vi "SLSC Scripting Constants.vi"() -> ()   [LabVIEW 2020, in "SLSC Switch Scripting.lvlib"]
doc: "Use this Global VI to access the GUIDs assigned to the page resources of the Custom Device."
uses:
  SLSC Switch Scripting.lvlib
panel:
  in  "Tab Control":T1(tab)=enum."Properties"
  in  "SLSC Sw:Status Section":string="Status"
  in  "SLSC Sw:Endpoint Section":string="Endpoint Configuration"
  in  "SLSC Sw:Prop:Reservation Group":string="Reservation Group"
  in  "SLSC Sw:Prop:Slot #":string="Slot #"
  in  "SLSC Sw:Prop:Model":string="Model"
  in  "SLSC Sw:Prop:Topology":string="Topology"
  in  "SLSC Sw:Prop:Switches JSON":string="Capabilities"
  in  "Compiled.Settings":string="Compiled.Settings"
  in  "GUID.SLSC Chassis":string="2d230194-1f79-4241-ad00-e5b0a0d634cb"
  in  "GUID.Status":string="fafe2633-52e8-4be6-bb95-b07e42834d60"
  in  "ChanList.HeartbeatChan":string="Heartbeat"
  in  "ChanList.StatusCode":string="Status code"
  in  "Desc.HeartbeatChan":string="Running count used for debugging. If this channel continues to increment, the custom device is still executing."
  in  "Desc.StatusCode":string="Status code of the custom device. A negative value indicates failure. A positive value indicates warning."
  in  "Paths.CDXML":path=path "SLSC Plugins/Modules/SLSC Switch/SLSC Module SLSC Switch.xml"
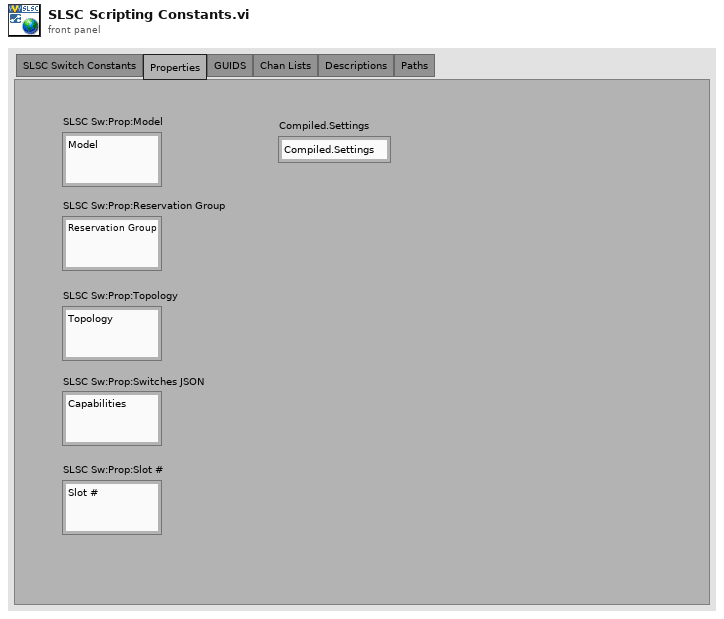
[diagram p1: front panel]
types:
  T1 = enum32{"SLSC Switch Constants", "Properties", "GUIDS", "Chan Lists", "Descriptions", "Paths"}
diagram:
